vi "SW_Globals.vi"() -> ()   [LabVIEW 2016]
panel:
  out "TTL recording start signal has been successfully reset":bool
  out "Recording has been started with TTL":bool
  out "Array of the presence count":u32[][](array[numeric])
  out "Active segments amount":u8
  out "Array of the segment to color correspondences":u32[][](array[numeric])
  out "Array of the pixel to color correspondences":u32[][](array[numeric])
  in  "Cluster of paths":T1
  out "Recording start timestamp":timestamp
  out "Color ramp array":u32[](array[colorbox])
  out "Diagram no zones":picture caption="Diagram at recording no zones"
  out "Diagram":picture
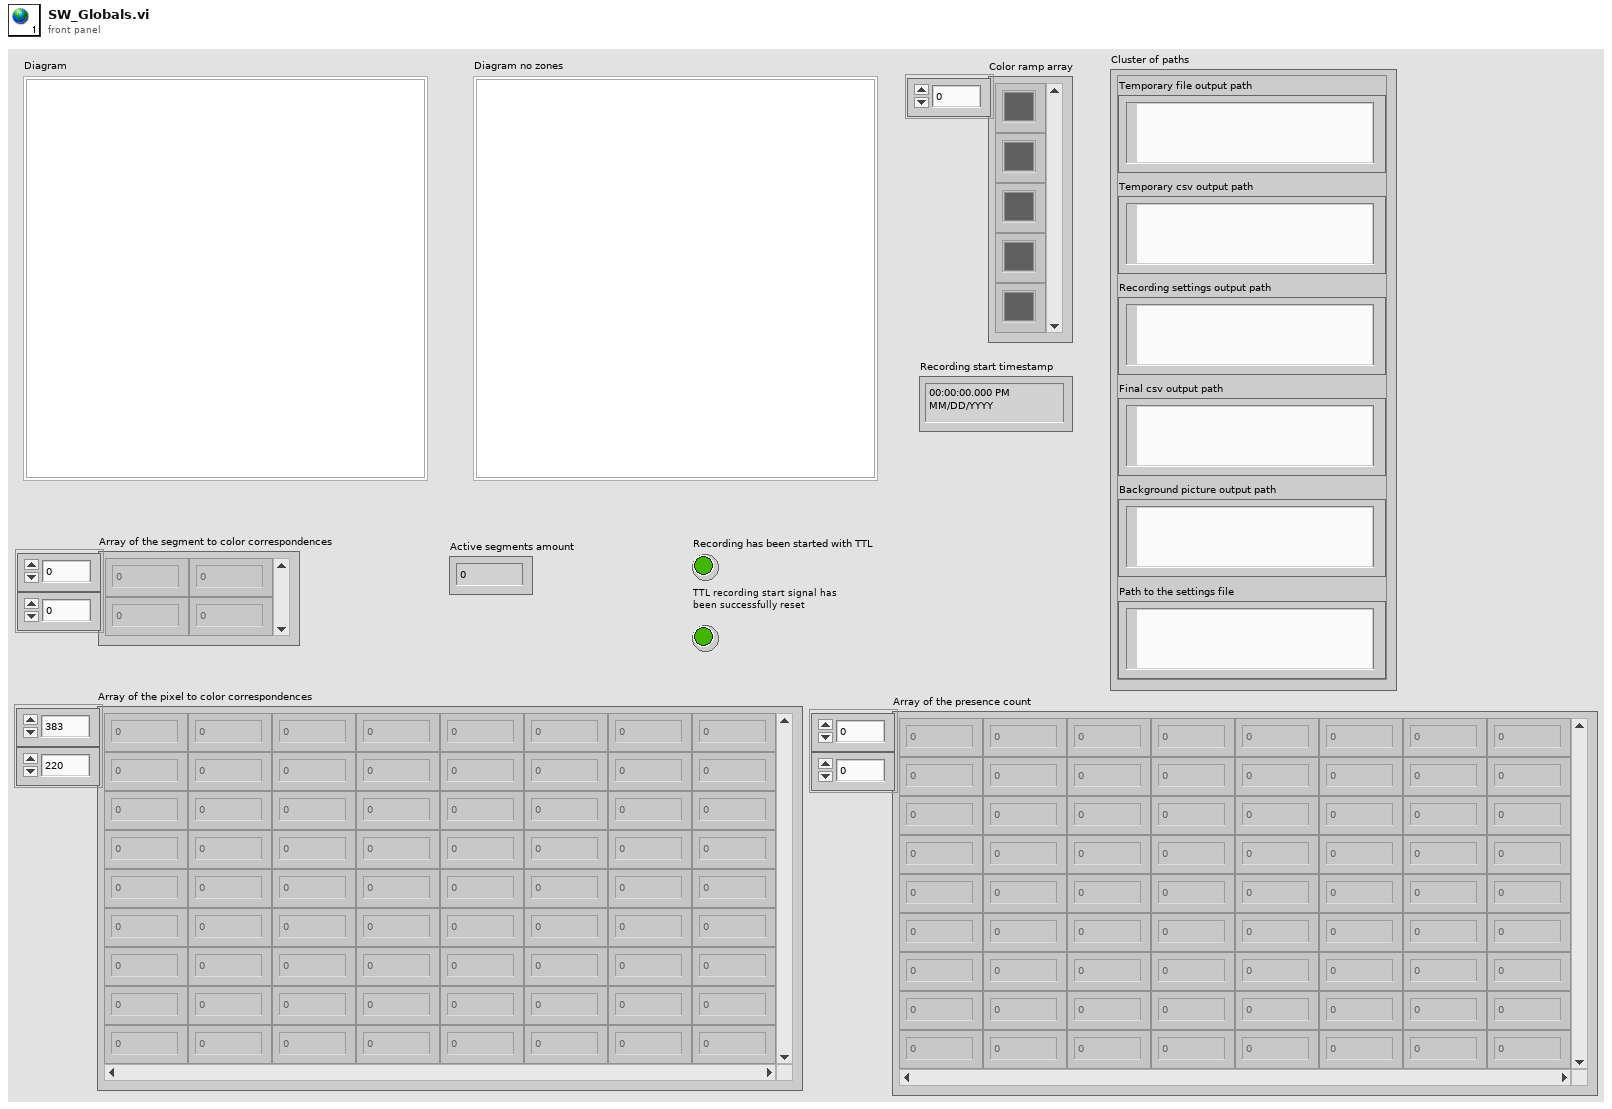
[diagram p1: front panel]
types:
  T1 = cluster{"Temporary file output path":path, "Temporary csv output path":path, "Recording settings output path":path, "Final csv output path":path, "Background picture output path":path, "Path to the settings file":path}
diagram:
